vi "ExScanSpectro.vi"() -> ()   [LabVIEW 2011]
panel:
  out "Current Wavelength":dbl format="%.2f"
  out "Scanning":bool
  in  "End Wavelength":dbl=700.0 format="%.2f"
  in  "Start Wavelength":dbl format="%.2f"
  in  "Scan Speed":dbl=2000.0 min=1.0 step=1.0 format="%.2f"
  in  "Grating number":i16=1 min=1 max=100 step=1
  out "error out":errorcluster
  in  "error in (no error)":errorcluster
  # "ExScanSpectro.vi\nThis VI is a simple example of how to setup and scan a spectrograph."
  # "NOTES:\nA properly configured spectometer .ini must be present in the LabVIEW folder for spectrograph operation.\n\nConsult the Toolkit documentation for more information on how to configure this file."
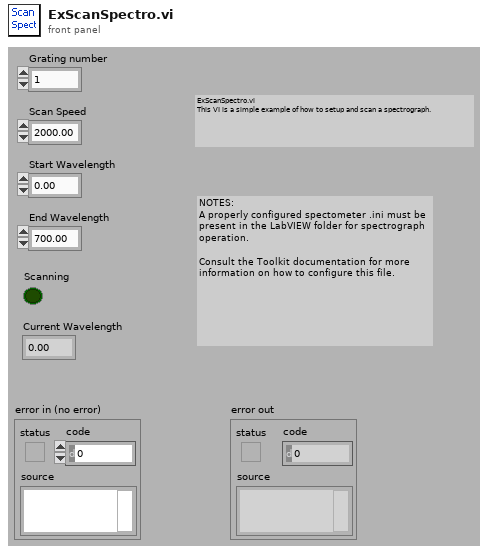
[diagram p1: front panel]
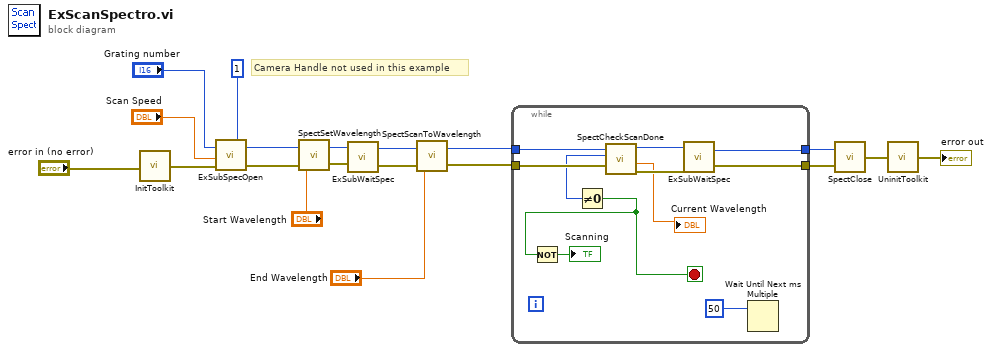
[diagram p0: block diagram]
diagram:
  # "Camera Handle not used in this example"
  n1 = call <userlib>:"InitToolkit.vi"("error in"="error in (no error)") -> ("error out"=w7:errorcluster)
  n2 = call "ExSubSpecOpen.vi"("error in (no error)"=w7, "Grating speed"="Scan Speed", "Grating number"="Grating number", "Camera Handles"=1) -> ("error out"=w13:errorcluster, "Spectrometer Handle"=w15:u32)  [unwired: 1 out]
  n3 = call <userlib>:"SpectSetWavelength.vi"("error in"=w13, "Wavelength"="Start Wavelength", "Spectrometer Handle"=w15) -> ("error out"=w17:errorcluster, "Spectrumeter Handle"=w16:u32)
  n4 = call "ExSubWaitSpec.vi"("error in (no error)"=w17, "Spectrometer Handle"=w16) -> ("error out"=w3:errorcluster, "Spectrometer handle"=w5:u32)
  n5 = call <userlib>:"SpectScanToWavelength.vi"("error in"=w3, "Wavelength"="End Wavelength", "Spectrometer Handle"=w5) -> ("error out"=w2:errorcluster, "Spectrometer Handle"=w4:u32)
  n6 = while {
    tunnel: w4 -> [w24]
    tunnel: [w28] -> w14
    tunnel: [w25] -> w12
    tunnel: w2 -> [w27]
    stop <- w21 stop-if-true
    n7 = call <userlib>:"SpectCheckScanDone.vi"("Spectrometer Handle"=w24, "error in"=w27) -> ("Spectrometer Handle"=w29:u32, "Done Flag"=w22:i16, "Wavelength"=→"Current Wavelength":dbl, "error out"=w26:errorcluster)
    n8 = Not Equal To 0?(x=w22) -> (x != 0?=w21:bool)
    n9 = Not(x=w21) -> (.not. x?=→"Scanning":bool)
    n10 = call "ExSubWaitSpec.vi"("error in (no error)"=w26, "Spectrometer Handle"=w29) -> ("error out"=w25:errorcluster, "Spectrometer handle"=w28:u32)
    n11 = Wait Until Next ms Multiple(millisecond multiple=50) -> ()  [unwired: 1 out]
  }
  n12 = call <userlib>:"SpectClose.vi"("error in"=w12, "Spectrometer Handle"=w14) -> ("error out"=w9:errorcluster)
  n13 = call <userlib>:"UninitToolkit.vi"("error in"=w9) -> ("error out"=→"error out":errorcluster)
